vi "UpdateImageInfo.vi"(0 "Image Refnum":refnum<vi>, 1 "Show Image Refnum":refnum<vi>, 2 "Isotropy (x/y) Refnum":refnum<vi>, 3 "operation":enum16{"set references", "update"}(ring)=enum."update") -> ()   [LabVIEW 2009]
uses:
  ImageSettings.ctt
  <vilib>/vision/Image Controls.llb/IMAQ Image.ctl
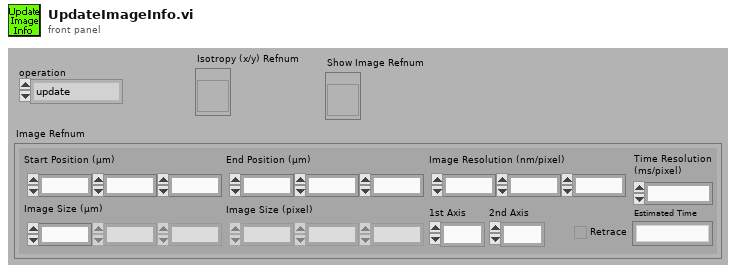
[diagram p1: front panel]
types:
  T1 = typedef "IMAQ Image.ctl" = refnum<image>
  T2 = typedef "DAQLinescanVisualization.ctt" = cluster{"Threshold":u32, "Trace Window #":u32, "IMAQ Trace":T1, "Retrace Window #":u32, "IMAQ Retrace":T1}
  T3 = cluster{"Start Position (µm)":cluster{"x":dbl, "y":dbl, "z":dbl}, "End Position (µm)":cluster{"x":dbl, "y":dbl, "z":dbl}, "Image Resolution (nm/pixel)":cluster{"x":dbl, "y":dbl, "z":dbl}, "Image Size (µm)":cluster{"x":dbl, "y":dbl, "z":dbl}, "Image Size (pixel)":cluster{"x":u32, "y":u32, "z":u32}, "Time Resolution\n(ms/pixel)":dbl, "1st Axis":u16, "2nd Axis":u16, "Retrace":bool, "Estimated Time":string}
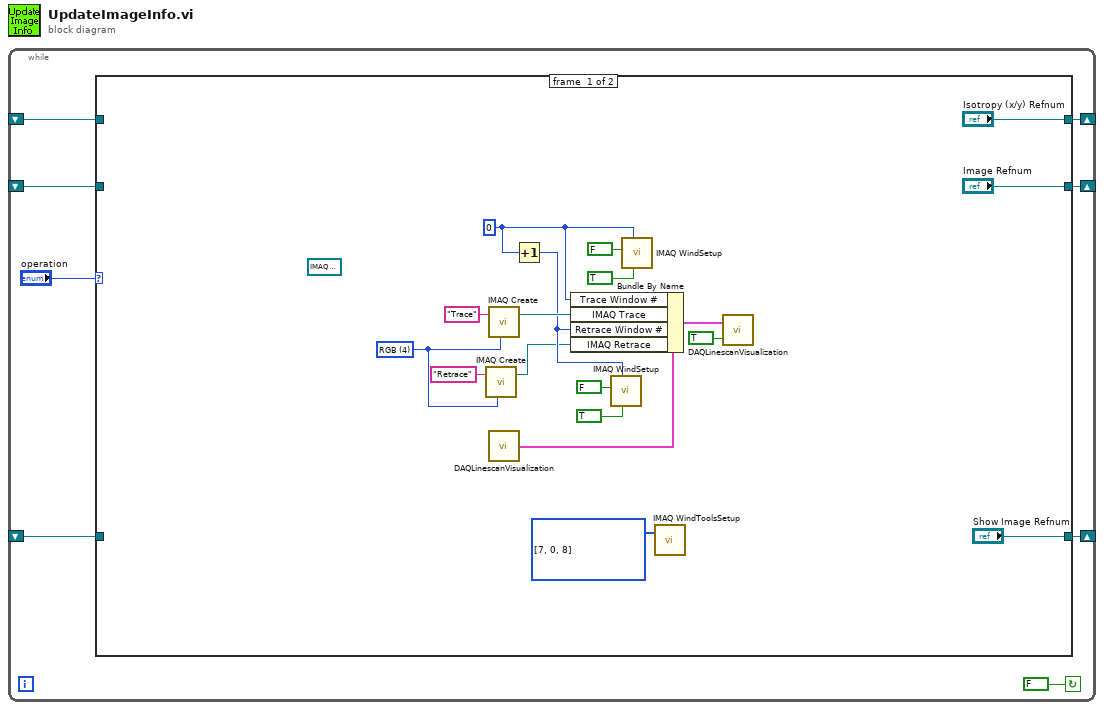
[diagram p0: block diagram]
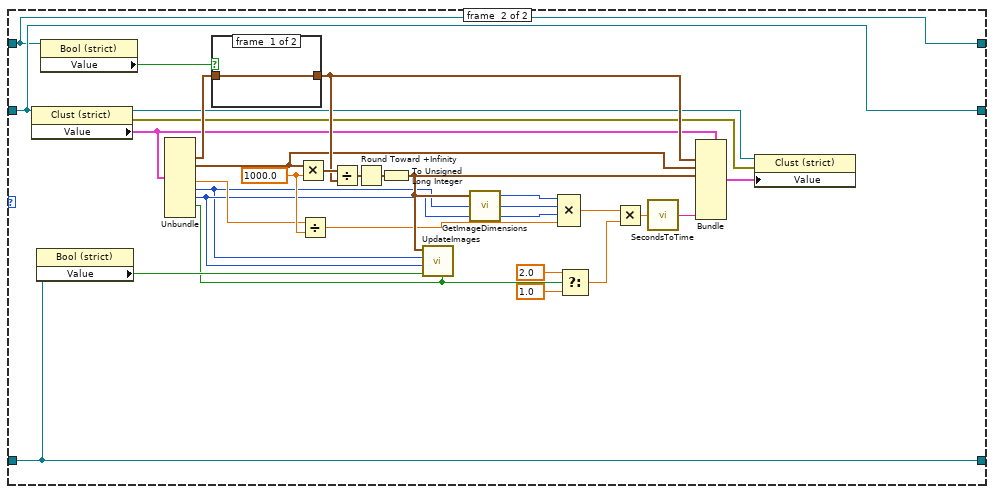
[diagram p2: hidden frame]
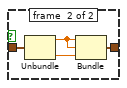
[diagram p3: hidden frame]
diagram:
  n1 = while {
    shift-right: [w5] -> _
    shift-left: _ -> [w6]
    shift-right: [w3] -> _
    shift-left: _ -> [w4]
    shift-right: [w1] -> _
    shift-left: _ -> [w2]
    stop <- FALSE continue-if-true
    n2 = case shown="\"set references\", Default" "operation" {
      tunnel: w6 -> [_ w44]
      tunnel: ["Image Refnum" w44] -> w5
      tunnel: w4 -> [_ w42]
      tunnel: ["Isotropy (x/y) Refnum" w42] -> w3
      tunnel: w2 -> [_ w41]
      tunnel: ["Show Image Refnum" w41] -> w1
      frame #0 {
        (unwired) T1 refnum ("New Image")
        w10 = u32[] [7, 0, 8] items=["Point", "Line", "Rectangle", "Oval", "Polygon", "Free", "Annulus", "Zoom", "Pan", "Broken Line", "Free Hand Line", "Rotated Rectangle"] ("Tools")
        w15 = u32 0 ("Window #")
        w13 = u32 4 items=["8 bits", "16 bits", "Float", "Complex", "RGB", "HSL"] ("Image Type")
        n3 = call "IMAQ Create"("Image Name"="Retrace", "Image Type"=w13) -> ("New Image"=w9:T1)  [unwired: 3 in, 1 out]
        n4 = call "IMAQ Create"("Image Name"="Trace", "Image Type"=w13) -> ("New Image"=w19:T1)  [unwired: 3 in, 1 out]
        n5 = call "DAQLinescanVisualization.vi"() -> ("Visualization (output)"=w11:T2)  [unwired: 2 in]
        n6 = Increment(x=w15) -> (x+1=w12:u32)
        n7 = Bundle By Name(cluster=w11, "Trace Window #"=w15, "IMAQ Trace"=w19, "Retrace Window #"=w12, "IMAQ Retrace"=w9) -> (w22:T2)
        n8 = call "IMAQ WindSetup"("Window is floating? (No)"=TRUE, "Window Number (0...15)"=w12, "Window can close? (Yes)"=FALSE) -> ()  [unwired: 8 in, 1 out]
        n9 = call "IMAQ WindSetup"("Window is floating? (No)"=TRUE, "Window Number (0...15)"=w15, "Window can close? (Yes)"=FALSE) -> ()  [unwired: 8 in, 1 out]
        n10 = call "IMAQ WindToolsSetup"("Tools"=w10) -> ()  [unwired: 5 in, 1 out]
        n11 = call "DAQLinescanVisualization.vi"("Get/Set"=TRUE, "Visualization (input)"=w22) -> ()  [unwired: 1 out]
      }
      frame #1 {
        w56 = 1000.0 ("y")
        n12 = property class="Clust (strict)"(reference=w44) -> (reference out=w50:refnum<vi>, error out=w49:errorcluster, "Value"=w51:T3)  [unwired: 1 in]
        n13 = property class="Bool (strict)"(reference=w41) -> ("Value"=w37:bool)  [unwired: 1 in, 2 out]
        n14 = property class="Bool (strict)"(reference=w42) -> ("Value"=w43:bool)  [unwired: 1 in, 2 out]
        n15 = Unbundle(w51) -> ("Image Resolution (nm/pixel)"=w53:cluster{"x":dbl, "y":dbl, "z":dbl}, "Image Size (µm)"=w47:cluster{"x":dbl, "y":dbl, "z":dbl}, "Time Resolution\n(ms/pixel)"=w54:dbl, "1st Axis"=w38:u16, "2nd Axis"=w39:u16, "Retrace"=w30:bool)  [unwired: 4 out]
        n16 = case shown="True" w43 {
          tunnel: w53 -> [w58 w61]
          tunnel: [w58 w60] -> w55
          frame #0 {
          }
          frame #1 {
            n17 = Unbundle(w61) -> ("x"=w62:dbl, "z"=w59:dbl)  [unwired: 1 out]
            n18 = Bundle("x"=w62, "x"=w62, "z"=w59) -> (w60:cluster{"x":dbl, "x":dbl, "z":dbl})  [unwired: 1 in]
          }
        }
        n19 = Multiply(x=w47, y=w56) -> (x*y=w57:cluster{"x":dbl, "y":dbl, "z":dbl})
        n20 = Divide(x=w54, y=w56) -> (x/y=w32:dbl)
        n21 = Divide(x=w57, y=w55) -> (x/y=w46:cluster{"x":dbl, dbl, "z":dbl})
        n22 = Round Toward +Infinity(x=w46) -> (ceil(x): smallest int >= x=w45:cluster{"x":dbl, dbl, "z":dbl})
        n23 = To Unsigned Long Integer(number=w45) -> (unsigned 32bit integer=w40:cluster{"x":u32, u32, "z":u32})
        n24 = call "UpdateImages.vi"("image size (pixel)"=w40, "1nd axis"=w38, "2nd axis"=w39, "show image"=w37, "retrace"=w30) -> ()  [unwired: 4 in]
        n25 = call "GetImageDimensions.vi"("2 nd Axis"=w39, "1st Axis"=w38, "Images Size (pixel)"=w40) -> ("planes"=w34:u32, "lines"=w35:u32, "columns"=w36:u32)
        n26 = Compound Arithmetic op=MULTIPLY(w36, w35, w34, w32) -> (w33:dbl)
        n27 = Select(t=2.0, s=w30, f=1.0) -> (s? t:f=w29:dbl)
        n28 = Multiply(x=w33, y=w29) -> (x*y=w31:dbl)
        n29 = call "SecondsToTime.vi"("Seconds"=w31) -> ("Time"=w52:string)
        n30 = Bundle(cluster=w51, "Image Resolution (nm/pixel)"=w55, "Image Size (µm)"=w47, "Image Size (pixel)"=w40, "Estimated Time"=w52) -> (w48:T3)  [unwired: 6 in]
        n31 = property class="Clust (strict)"(reference=w50, error in=w49, "Value"=w48) -> ()  [unwired: 2 out]
      }
    }
  }
